vi "Compiled Get Sim Device Settings.vi"(8 "error in (no error)":errorcluster, 9 "Database Ref":refnum<k21>, 11 "Addon Ref":T1 format="%.0x") -> (0 "error out":errorcluster, 2 "Settings":T2[](array[typedef]) {"DTCs"."DM1.Ref"."Data Reference" format="%.0x"; "DTCs"."DM1.Enable.Ref"."Data Reference" format="%.0x"; "DTCs"."DM2.Ref"."Data Reference" format="%.0x"; "DTCs"."DM2.Enable.Ref"."Data Reference" format="%.0x"; "Data"."Outgoing"."Trigger.Refs"."Data Reference" format="%.0x"; "Data"."Outgoing"."Disable.Refs"."Data Reference" format="%.0x"; "Data"."Outgoing"."Data.Refs"."Data Reference" format="%.0x"; "Data"."Incoming"."Timing.Refs"."Data Reference" format="%.0x"; "Data"."Incoming"."Data.Refs"."Data Reference" format="%.0x"; "Network"."Name" format="%.0x"}, 3 "Addon Ref out":T1 format="%.0x")   [LabVIEW 2015, in "J1939 Addon System Explorer.lvlib"]
uses:
  J1939 Addon System Explorer.lvlib
  <vilib>/NI Veristand/Custom Device API/Custom Device Item Ref.ctl
  Shared/Types/Complied Simulated Device Settings.ctl
  Shared/Types/Monitor Settings.ctl
  Shared/Types/Device Settings.ctl
  Shared/Types/Incoming Settings.ctl
  Shared/Types/Frame Settings.ctl
  Shared/Types/Outgoing Event Trigger Types.ctl
  <vilib>/NI Veristand/Custom Device API/Block Data Reference.ctl
  <vilib>/NI Veristand/Custom Device API/Data Reference.ctl
  Shared/Types/Outgoing Settings.ctl
  Shared/Types/Compiled Simulated Settings.ctl
  <vilib>/NI Veristand/Custom Device Tools/Custom Device Utility Library/NI VeriStand - Search for All Items by GUID.vi
  Shared/SubVIs/Constants.vi
  <vilib>/NI VeriStand/Custom Device Tools/Custom Device Utility Library/Custom Device Utility Library.lvlib
  Shared/J1939 Addon Shared.lvlib
  <vilib>/NI VeriStand/Custom Device API/Custom Device API.lvlib
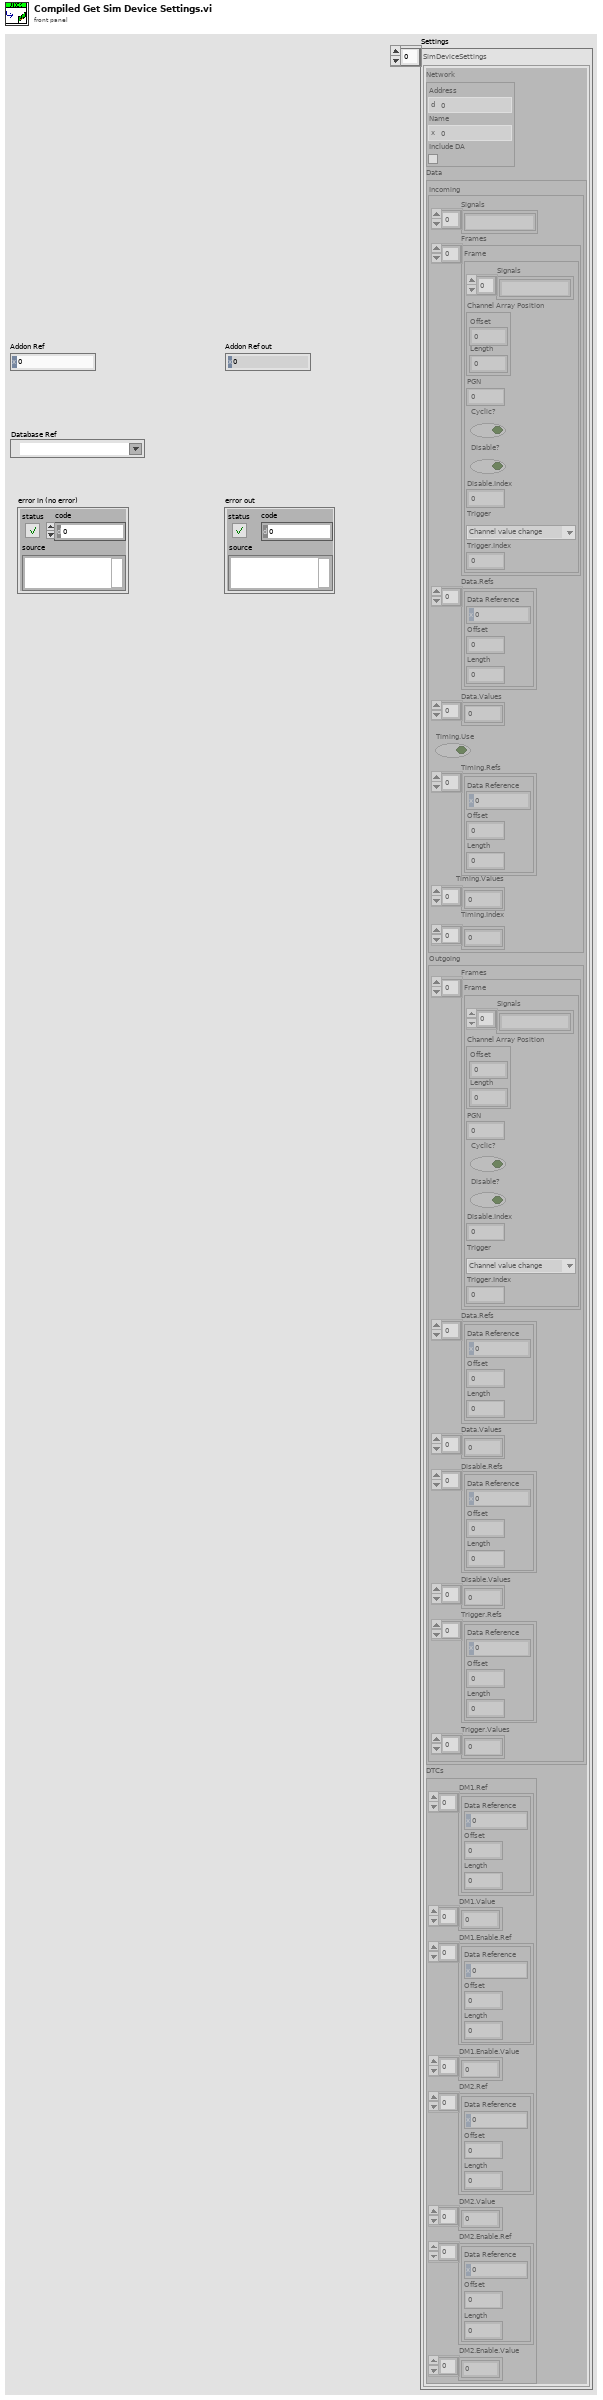
[diagram p1: front panel]
types:
  T1 = typedef "Custom Device API.lvlib/Custom Device Item Ref.ctl" = u64
  T2 = typedef "J1939 Addon Shared.lvlib/Complied Simulated Device Settings.ctl" = cluster{"Network":T3, "Data":T4, "DTCs":T11}
  T3 = typedef "J1939 Addon Shared.lvlib/Monitor Settings.ctl" = cluster{"Address":u8, "Name":u64, "Include DA":bool}
  T4 = typedef "J1939 Addon Shared.lvlib/Device Settings.ctl" = cluster{"Incoming":T5, "Outgoing":T10}
  T5 = typedef "J1939 Addon Shared.lvlib/Incoming Settings.ctl" = cluster{"Signals":string[], "Frames":T6[], "Data.Refs":T8[], "Data.Values":dbl[], "Timing.Use":bool, "Timing.Refs":T8[], "Timing.Values":dbl[], "Timing.Index":i32[]}
  T6 = typedef "J1939 Addon Shared.lvlib/Frame Settings.ctl" = cluster{"Signals":string[], "Channel Array Position":cluster{"Offset":u32, "Length":u32}, "PGN":u32, "Cyclic?":bool, "Disable?":bool, "Disable.Index":i32, "Trigger":T7, "Trigger.Index":i32}
  T7 = typedef "J1939 Addon Shared.lvlib/Outgoing Event Trigger Types.ctl" = enum16{"Channel value change", "Trigger channel (not zero)", "Channel value change or trigger channel (not zero)", "Trigger channel (any value change)", "Channel value change or trigger channel (any value change)"}
  T8 = typedef "Custom Device API.lvlib/Block Data Reference.ctl" = cluster{"Data Reference":T9, "Offset":u64, "Length":u64}
  T9 = typedef "Custom Device API.lvlib/Data Reference.ctl" = i32
  T10 = typedef "J1939 Addon Shared.lvlib/Outgoing Settings.ctl" = cluster{"Frames":T6[], "Data.Refs":T8[], "Data.Values":dbl[], "Disable.Refs":T8[], "Disable.Values":dbl[], "Trigger.Refs":T8[], "Trigger.Values":dbl[]}
  T11 = typedef "J1939 Addon Shared.lvlib/Compiled Simulated Settings.ctl" = cluster{"DM1.Ref":T8[], "DM1.Value":dbl[], "DM1.Enable.Ref":T8[], "DM1.Enable.Value":dbl[], "DM2.Ref":T8[], "DM2.Value":dbl[], "DM2.Enable.Ref":T8[], "DM2.Enable.Value":dbl[]}
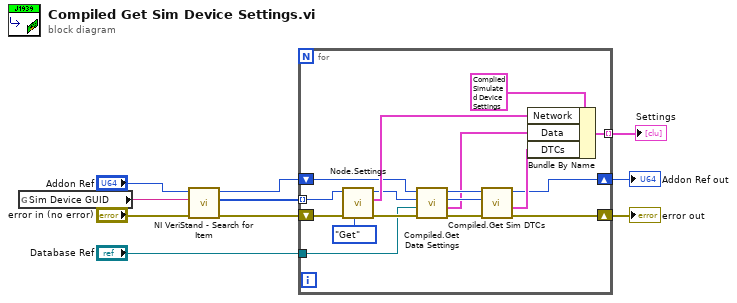
[diagram p0: block diagram]
diagram:
  n1 = global read "Constants.vi" "Sim Device GUID"() -> (w1:string)
  n2 = call-poly <vilib>:"NI VeriStand - Search for Item.vi"("error in"="error in (no error)", "Item GUID"=w1, "Section Ref in"="Addon Ref") -> ("error out"=w3:errorcluster, "Item Refs"=w4:T1[], "Section Ref out"=w7:T1)  [unwired: 5 in, 1 out]
  n3 = for {
    tunnel: w4 -> [w26] mode=indexing
    shift-right: [w12] -> w10
    shift-left: w7 -> [w18]
    shift-right: [w20] -> w8
    shift-left: w3 -> [w27]
    tunnel: "Database Ref" -> [w19]
    tunnel: [w22] -> w2 mode=indexing
    n4 = call "Node.Settings.vi"("Action"=enum8{"Get", "Set"}."Get", "error in (no error)"=w27, "Item Ref in"=w26) -> ("error out"=w25:errorcluster, "Node.Settings"=w23:T3, "Item Ref out"=w16:T1)  [unwired: 6 in]
    n5 = call "Compiled.Get Data Settings.vi"("error in (no error)"=w25, "Database Ref"=w19, "Node Ref in"=w16, "Addon Ref In"=w18) -> ("error out"=w21:errorcluster, "Node Data Refs"=w14:T4, "Node Ref out"=w15:T1, "Addon Ref out"=w17:T1)  [unwired: 4 in]
    n6 = call "Compiled.Get Sim DTCs.vi"("error in (no error)"=w21, "Node Ref in"=w15, "Addon Ref in"=w17) -> ("error out"=w20:errorcluster, "Sim DTCs"=w13:T11, "Addon Ref out"=w12:T1)  [unwired: 5 in, 1 out]
    n7 = Bundle By Name(cluster=T2 {"Network"={"Address"=0, "Name"=0, "Include DA"=FALSE}, "Data"={"Incoming"={"Signals"=[], "Frames"=[], "Data.Refs"=[], "Data.Values"=[], "Timing.Use"=FALSE, "Timing.Refs"=[], "Timing.Values"=[], "Timing.Index"=[]}, "Outgoing"={"Frames"=[], "Data.Refs"=[], "Data.Values"=[], "Disable.Refs"=[], "Disable.Values"=[], "Trigger.Refs"=[], "Trigger.Values"=[]}}, "DTCs"={"DM1.Ref"=[], "DM1.Value"=[], "DM1.Enable.Ref"=[], "DM1.Enable.Value"=[], "DM2.Ref"=[], "DM2.Value"=[], "DM2.Enable.Ref"=[], "DM2.Enable.Value"=[]}} ("SimDeviceSettings"), "Network"=w23, "Data"=w14, "DTCs"=w13) -> (w22:T2)
  }
  "Addon Ref out" <- w10
  "Settings" <- w2
  "error out" <- w8
